vi "config Spark Max.vi"(5 "Reverse Limit switch":T1=enum."Normally Closed", 6 "LIMIT SW\nEnabled?":bool, 7 "Forward Limit switch":T1=enum."Normally Closed", 8 "error in (no error)":errorcluster, 11 "motor\ndefaults":T2={"description"="", "MOTOR SELECT"=0, "Installed?"=FALSE, "CAN ID"=0, "refnum name"="", "Invert"=FALSE, "Idle Mode"=enum."Coast", "Current limiting"={"Linearized"=FALSE, "Free Speed (A)"=0.0, "Primay (A)"=0.0, "Limit RPM (0)"=0}, "MOTOR PIDF coefficients"={"PIDF"={"P Gain"=0.001, "I Gain"=0.0, "D Gain"=0.0, "F Gain"=0.0012, "I Zone"=0.0, "Min Output"=-1.0, "Max Output"=1.0}, "Smart Motion"={"Max Velocity"=1900.0, "Max Acceleration"=750.0, "Minimum Velocity Output"=0.1, "Allowed Closed Loop Error"=0.02}}, "gear ratio"=0.0} {"gear ratio" format="%_5f"; "MOTOR SELECT" items=["REV NEO"=5676, "REV NEO 550"=11000, "VEX Falcon"=6380, "WC Kraken"=6000]}) -> (0 "error out":errorcluster, 3 "MotorControlDevRef":T8)   [LabVIEW 2023]
uses:
  <vilib>/Rock Robotics/WPI/MotorControl/WPI_MotorControlDeviceRef.ctl
  <vilib>/Rock Robotics/WPI/MotorControl/WPI_MotorControlType.ctl
  <vilib>/Rock Robotics/SystemInterfaces/DIO/FPGA_DIOPWMChannel.ctl
  <vilib>/Rock Robotics/WPI/PWM/WPI_PWMDeadband.ctl
  <vilib>/Rock Robotics/SystemInterfaces/DIO/FPGA_DIOChannel.ctl
  ctrl defs/ctrl swerve motor.ctl
  ctrl defs/ctrl MOTOR SELECT.ctl
  <vilib>/Rock Robotics/WPI/ThirdParty/REV Robotics/REVLib/Typedef/Spark MAX Idle Mode.ctl
  ctrl defs/ctrl Spark MAX current limiting.ctl
  ctrl defs/ctrl motor PIDF coefficients.ctl
  <vilib>/Rock Robotics/WPI/ThirdParty/REV Robotics/REVLib/Typedef/Spark MAX Smart Motion Parameters.ctl
  <vilib>/Rock Robotics/WPI/ThirdParty/REV Robotics/REVLib/Typedef/Spark MAX Limit Switch Polarity.ctl
  <vilib>/Rock Robotics/WPI/ThirdParty/REV Robotics/REVLib/Typedef/Spark MAX Motor Type.ctl
  <vilib>/Rock Robotics/WPI/ThirdParty/REV Robotics/REVLib/Typedef/Spark MAX Sensor Type.ctl
  <vilib>/Rock Robotics/WPI/ThirdParty/REV Robotics/REVLib/Typedef/Spark MAX Limit Direction.ctl
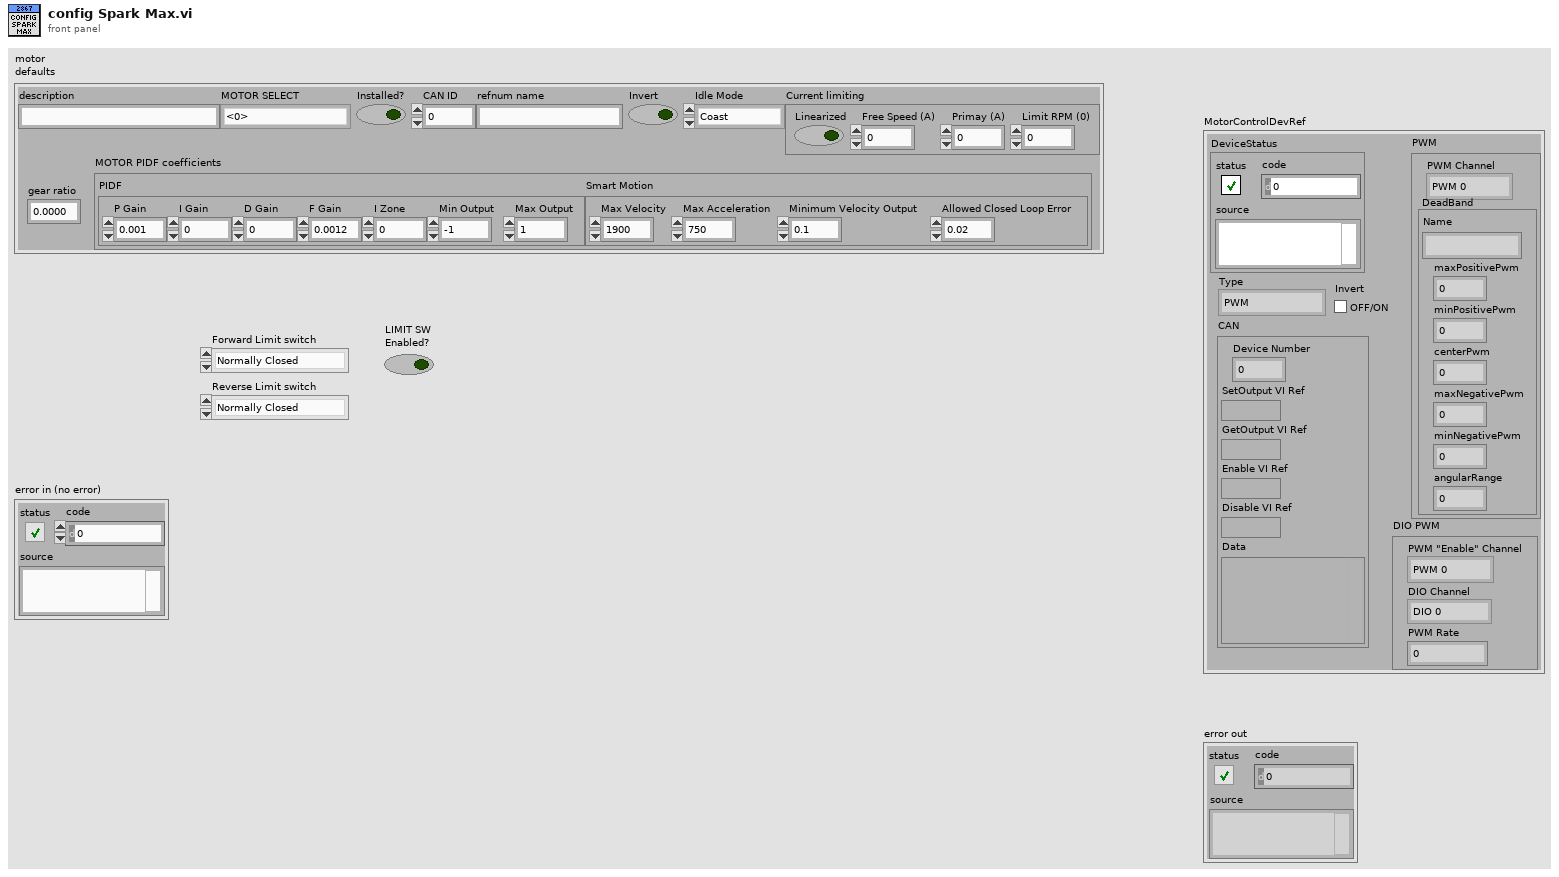
[diagram p1: front panel]
types:
  T1 = typedef "Spark MAX Limit Switch Polarity.ctl" = enum16{"Normally Open", "Normally Closed"}
  T2 = typedef "ctrl swerve motor.ctl" = cluster{"description":string, "MOTOR SELECT":T3, "Installed?":bool, "CAN ID":u8, "refnum name":string, "Invert":bool, "Idle Mode":T4, "Current limiting":T5, "MOTOR PIDF coefficients":T6, "gear ratio":dbl}
  T3 = typedef "ctrl MOTOR SELECT.ctl" = i16
  T4 = typedef "Spark MAX Idle Mode.ctl" = enum16{"Coast", "Brake"}
  T5 = typedef "ctrl Spark MAX current limiting.ctl" = cluster{"Linearized":bool, "Free Speed (A)":dbl, "Primay (A)":dbl, "Limit RPM (0)":u32}
  T6 = typedef "ctrl motor PIDF coefficients.ctl" = cluster{"PIDF":cluster{"P Gain":dbl, "I Gain":dbl, "D Gain":dbl, "F Gain":dbl, "I Zone":dbl, "Min Output":dbl, "Max Output":dbl}, "Smart Motion":T7}
  T7 = typedef "Spark MAX Smart Motion Parameters.ctl" = cluster{"Max Velocity":dbl, "Max Acceleration":dbl, "Minimum Velocity Output":dbl, "Allowed Closed Loop Error":dbl}
  T8 = typedef "WPI_MotorControlDeviceRef.ctl" = cluster{"DeviceStatus":errorcluster, "Type":T9, "PWM":cluster{"PWM Channel":T10, "DeadBand":T11}, "CAN":cluster{"Device Number":u8, "SetOutput VI Ref":variant, "GetOutput VI Ref":variant, "Enable VI Ref":variant, "Disable VI Ref":variant, "Data":variant}, "Invert":bool, "DIO PWM":cluster{"PWM \"Enable\" Channel":T10, "DIOChannel":T12, "PWM Rate":dbl}}
  T9 = typedef "WPI_MotorControlType.ctl" = enum16{"PWM", "CAN", "DIO PWM"}
  T10 = typedef "FPGA_DIOPWMChannel.ctl" = enum8{"PWM 0", "PWM 1", "PWM 2", "PWM 3", "PWM 4", "PWM 5", "PWM 6", "PWM 7", "PWM 8", "PWM 9", "PWM MXP 0", "PWM MXP 1", "PWM MXP 2", "PWM MXP 3", "PWM MXP 4", "PWM MXP 5", "PWM MXP 6", "PWM MXP 7", "PWM MXP 8", "PWM MXP 9", "Invalid"}
  T11 = typedef "WPI_PWMDeadband.ctl" = cluster{"Name":string, "maxPositivePwm":i32, "minPositivePwm":i32, "centerPwm":i32, "maxNegativePwm":i32, "minNegativePwm":i32, "angularRange":u16}
  T12 = typedef "FPGA_DIOChannel.ctl" = enum8{"DIO 0", "DIO 1", "DIO 2", "DIO 3", "DIO 4", "DIO 5", "DIO 6", "DIO 7", "DIO 8", "DIO 9", "DIO MXP 0", "DIO MXP 1", "DIO MXP 2", "DIO MXP 3", "DIO MXP 4", "DIO MXP 5", "DIO MXP 6", "DIO MXP 7", "DIO MXP 8", "DIO MXP 9", "DIO MXP 10", "DIO MXP 11", "DIO MXP 12", "DIO MXP 13", "DIO MXP 14", "DIO MXP 15", "SPI Port CS1", "SPI Port CS2", "SPI Port CS3", "SPI Port MISO", "SPI Port MOSI", "Invalid"}
  T13 = typedef "Spark MAX Motor Type.ctl" = enum16{"Brushed", "Brushless"}
  T14 = typedef "Spark MAX Sensor Type.ctl" = enum16{"No Sensor", "Hall Sensor", "Encoder", "-Not Available-", "Analog", "Alternate Encoder", "Duty Cycle"}
  T15 = typedef "Spark MAX Limit Direction.ctl" = enum16{"Forward Limit", "Reverse Limit"}
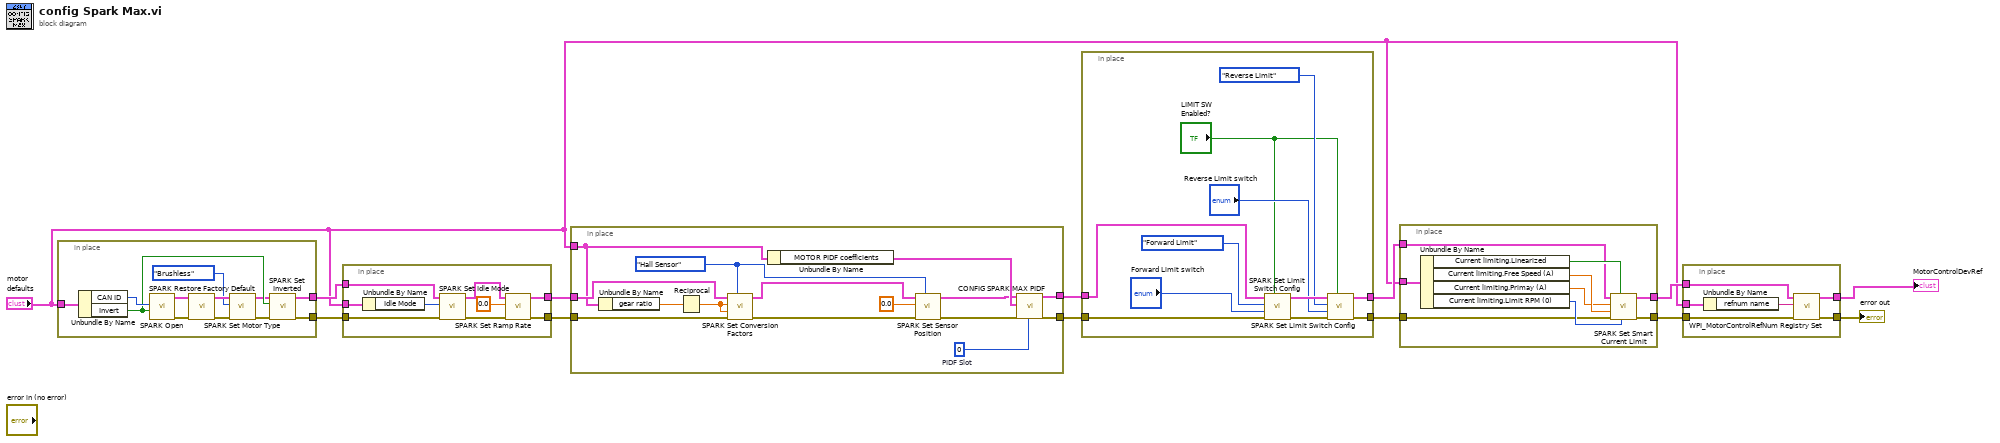
[diagram p0: block diagram]
diagram:
  n1 = in-place {
    in-place-border: [w23] -> w9
    in-place-border: [w22] -> w8
    in-place-border: "motor\ndefaults" -> [w18]
    n2 = Unbundle By Name(w18) -> ("CAN ID"=w25:u8, "Invert"=w24:bool)
    n3 = call <vilib>:"SPARK Open.vi"("Invert"=w24, "Device Number"=w25) -> ("error out"=w19:errorcluster, "MotorControlDeviceRef"=w20:T8)  [unwired: 8 in]
    n4 = call <vilib>:"SPARK Restore Factory Default.vi"("error in"=w19, "MotorControlDeviceRef"=w20) -> ("error out"=w16:errorcluster, "MotorControlDeviceRef"=w21:T8)  [unwired: 8 in]
    n5 = call <vilib>:"SPARK Set Motor Type.vi"("error in (no error)"=w16, "Motor Type"=Spark_MAX_Motor_Type."Brushless", "MotorControlDevRef"=w21) -> ("error out"=w15:errorcluster, "MotorControlDeviceRef"=w17:T8)  [unwired: 7 in]
    n6 = call <vilib>:"SPARK Set Inverted.vi"("error in (no error)"=w15, "Inverted (F)"=w24, "MotorControlDeviceRef in"=w17) -> ("error out"=w23:errorcluster, "MotorControlDeviceRef out"=w22:T8)  [unwired: 7 in]
  }
  n7 = in-place {
    in-place-border: w9 -> [w34]
    in-place-border: w8 -> [w33]
    in-place-border: [w29] -> w4
    in-place-border: [w27] -> w5
    in-place-border: "motor\ndefaults" -> [w30]
    n8 = Unbundle By Name(w30) -> ("Idle Mode"=w31:T4)
    n9 = call <vilib>:"SPARK Set Idle Mode.vi"("error in (no error)"=w34, "Idle Mode"=w31, "MotorControlDeviceRef in"=w33) -> ("error out"=w28:errorcluster, "MotorControlDeviceRef out"=w32:T8)  [unwired: 7 in]
    n10 = call <vilib>:"SPARK Set Ramp Rate.vi"("error in (no error)"=w28, "Seconds from neutral to full (0)"=sgl 0.0, "MotorControlDeviceRef in"=w32) -> ("error out"=w27:errorcluster, "MotorControlDeviceRef"=w29:T8)  [unwired: 7 in]
  }
  n11 = in-place {
    in-place-border: w5 -> [w49]
    in-place-border: w4 -> [w48]
    in-place-border: [w44] -> w3
    in-place-border: [w43] -> w2
    in-place-border: "motor\ndefaults" -> [w42]
    w40 = 0  # PIDF Slot
    w38 = Spark_MAX_Sensor_Type."Hall Sensor" ("Sensor Type (Hall Sensor)")
    n12 = Unbundle By Name(w42) -> ("gear ratio"=w47:dbl)
    n13 = Reciprocal(x=w47) -> (1/x=w46:dbl)
    n14 = call <vilib>:"SPARK Set Conversion Factors.vi"("Sensor Type (Hall Sensor)"=w38, "error in (no error)"=w49, "Velocity Factor (1)"=w46, "Position Factor (1)"=w46, "MotorControlDeviceRef in"=w48) -> ("error out"=w36:errorcluster, "MotorControlDeviceRef out"=w45:T8)  [unwired: 5 in]
    n15 = Unbundle By Name(w42) -> ("MOTOR PIDF coefficients"=w41:T6)
    n16 = call <vilib>:"SPARK Set Sensor Position.vi"("Sensor Type (Hall Sensor)"=w38, "error in"=w36, "Position"=0.0, "MotorControlDeviceRef"=w45) -> ("error out"=w35:errorcluster, "MotorControlDeviceRef"=w39:T8)  [unwired: 6 in]
    n17 = call "CONFIG SPARK MAX PIDF.vi"("MotorControlDevRef"=w39, "MOTOR PIDF coefficients"=w41, "error in (no error)"=w35, "PIDF Slot"=w40) -> ("MotorControlDevRef OUT"=w44:T8, "error out"=w43:errorcluster)  [unwired: 14 in]
  }
  n18 = in-place {
    in-place-border: w3 -> [w60]
    in-place-border: [w57] -> w7
    in-place-border: w2 -> [w54]
    in-place-border: [w52] -> w6
    n19 = call <vilib>:"SPARK Set Limit Switch Config.vi"("Enabled? (T)"="LIMIT SW\nEnabled?", "error in (no error)"=w54, "Polarity (Normally Open)"="Forward Limit switch", "Limit Switch"=Spark_MAX_Limit_Direction."Forward Limit", "MotorControlDeviceRef in"=w60) -> ("error out"=w53:errorcluster, "MotorControlDeviceRef out"=w59:T8)  [unwired: 5 in]
    n20 = call <vilib>:"SPARK Set Limit Switch Config.vi"("Enabled? (T)"="LIMIT SW\nEnabled?", "error in (no error)"=w53, "Polarity (Normally Open)"="Reverse Limit switch", "Limit Switch"=Spark_MAX_Limit_Direction."Reverse Limit", "MotorControlDeviceRef in"=w59) -> ("error out"=w52:errorcluster, "MotorControlDeviceRef out"=w57:T8)  [unwired: 5 in]
  }
  n21 = in-place {
    in-place-border: [w69] -> w12
    in-place-border: [w64] -> w10
    in-place-border: w7 -> [w63]
    in-place-border: w6 -> [w62]
    in-place-border: "motor\ndefaults" -> [w61]
    n22 = Unbundle By Name(w61) -> ("Current limiting.Linearized"=w65:bool, "Current limiting.Free Speed (A)"=w67:dbl, "Current limiting.Primay (A)"=w66:dbl, "Current limiting.Limit RPM (0)"=w68:u32)
    n23 = call <vilib>:"SPARK Set Smart Current Limit.vi"("Linear Limit RPM (0)"=w68, "Linearized Limit Enabled (F)"=w65, "error in (no error)"=w62, "Free Speed Current Limit (20A)"=w67, "Primay Current Limit (80A)"=w66, "MotorControlDeviceRef in"=w63) -> ("error out"=w69:errorcluster, "MotorControlDeviceRef out"=w64:T8)  [unwired: 4 in]
  }
  n24 = in-place {
    in-place-border: [w75] -> w13
    in-place-border: w12 -> [w74]
    in-place-border: [w73] -> w11
    in-place-border: w10 -> [w72]
    in-place-border: "motor\ndefaults" -> [w70]
    n25 = Unbundle By Name(w70) -> ("refnum name"=w71:string)
    n26 = call <vilib>:"WPI_MotorControlRefNum Registry Set.vi"("error in (no error)"=w74, "refnum name"=w71, "MotorControlDevRef"=w72) -> ("error out"=w75:errorcluster, "MotorControlDevRef"=w73:T8)  [unwired: 7 in]
  }
  "error out" <- w13
  "MotorControlDevRef" <- w11
